vi "Run Caliper.vi"(6 "SelectionList":T3[](array[typedef]), 8 "error in (no error)":errorcluster, 9 "FilteredCaliperEntry":T6[](array[typedef]) {"CaliperType" items=["Distance", "Mid Point", "Perpendicular Projection", "Lines Intersection", "Angle from Horizontal", "Angle from Vertical", "Angle Defined by 3 Points", "Angle Defined by 4 Points", "Bissecting Line", "Mid Line", "Center of Mass", "Area", "Line Fit", "Circle Fit", "Ellipse Fit"]}, 10 "Analysis_Point_Result":T8[](array[typedef]), 11 "CaliperType":T2 items=["Distance", "Mid Point", "Perpendicular Projection", "Lines Intersection", "Angle from Horizontal", "Angle from Vertical", "Angle Defined by 3 Points", "Angle Defined by 4 Points", "Bissecting Line", "Mid Line", "Area", "Line Fit", "Circle Fit"]) -> (0 "error out":errorcluster, 2 "SelectionListOut":T3[](array[typedef]), 3 "Result":T5)   [LabVIEW 2019]
uses:
  Controls/CaliperType.ctl
  Controls/SelectionListEntry.ctl
  Controls/SelectionListEntryPointType.ctl
  Analysis/Controls/Analysis_Result_To_Caliper.ctl
  Controls/CaliperDataEntry_SinglePoint.ctl
  Controls/CaliperResult_SinglePoint.ctl
  Controls/CaliperResult.ctl
  Controls/CaliperDataEntry.ctl
  <vilib>/vision/NI_Vision_Development_Module.lvlib
panel:
  in  "CaliperEntry 2":T1 {"CaliperType" items=["Distance", "Mid Point", "Perpendicular Projection", "Lines Intersection", "Angle from Horizontal", "Angle from Vertical", "Angle Defined by 3 Points", "Angle Defined by 4 Points", "Bissecting Line", "Mid Line", "Center of Mass", "Area", "Line Fit", "Circle Fit", "Ellipse Fit"]}
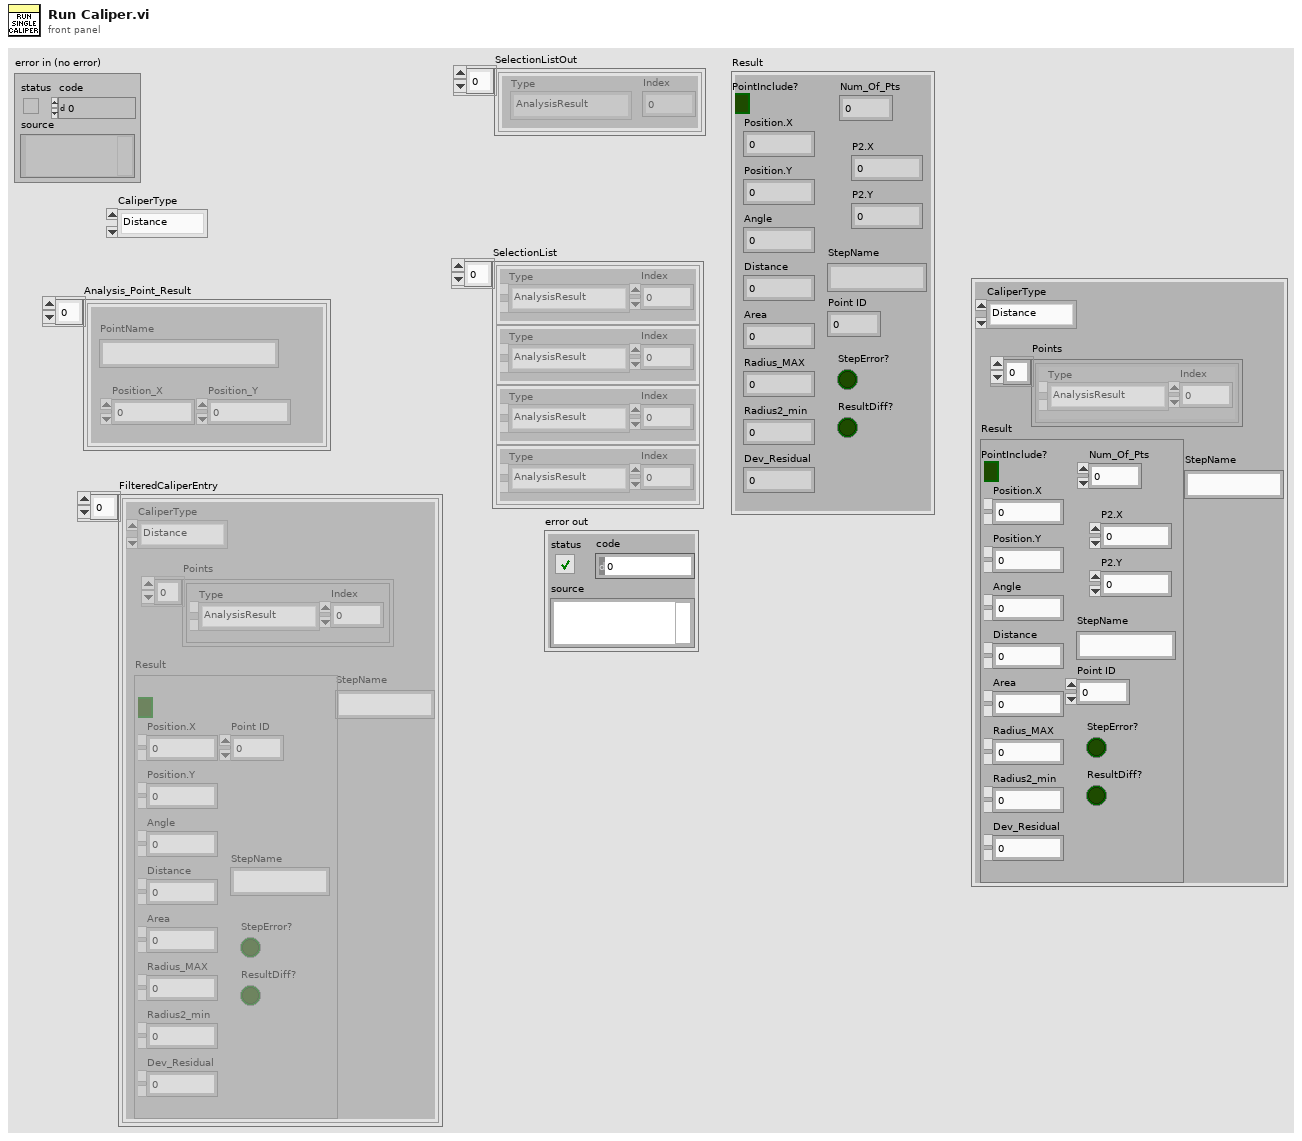
[diagram p1: front panel]
types:
  T1 = typedef "CaliperDataEntry.ctl" = cluster{"CaliperType":T2, "Points":T3[], "Result":T5, "StepName":string}
  T2 = typedef "CaliperType.ctl" = u32
  T3 = typedef "SelectionListEntry.ctl" = cluster{"Type":T4, "Index":i32}
  T4 = typedef "SelectionListEntryPointType.ctl" = enum16{"AnalysisResult", "CaliperResult"}
  T5 = typedef "CaliperResult.ctl" = cluster{"PointInclude?":bool, "Num_Of_Pts":u8, "Position.X":dbl, "Position.Y":dbl, "Angle":dbl, "Distance":dbl, "Area":dbl, "Radius_MAX":dbl, "Radius2_min":dbl, "Dev_Residual":dbl, "P2.X":dbl, "P2.Y":dbl, "StepName":string, "Point ID":u8, "StepError?":bool, "ResultDiff?":bool}
  T6 = typedef "CaliperDataEntry_SinglePoint.ctl" = cluster{"CaliperType":T2, "Points":T3[], "Result":T7, "StepName":string}
  T7 = typedef "CaliperResult_SinglePoint.ctl" = cluster{"PointInclude?":bool, "Position.X":dbl, "Position.Y":dbl, "Angle":dbl, "Distance":dbl, "Area":dbl, "Radius_MAX":dbl, "Radius2_min":dbl, "Dev_Residual":dbl, "StepName":string, "Point ID":u8, "StepError?":bool, "ResultDiff?":bool}
  T8 = typedef "Analysis_Result_To_Caliper.ctl" = cluster{"PointName":string, "Position_X":dbl, "Position_Y":dbl}
  T9 = cluster{cluster{"Position.X":dbl, "Position.Y":dbl}, cluster{"Position.X":dbl, "Position.Y":dbl}}
  T10 = cluster{"Point 1":cluster{"X":sgl, "Y":sgl}, "Point 2":cluster{"X":sgl, "Y":sgl}}
  T11 = cluster{"element":cluster{"Position_X":dbl, "Position_Y":dbl}, "element":cluster{"Position_X":dbl, "Position_Y":dbl}}
  T12 = cluster{"Center":cluster{"X":sgl, "Y":sgl}, "Radius":dbl}
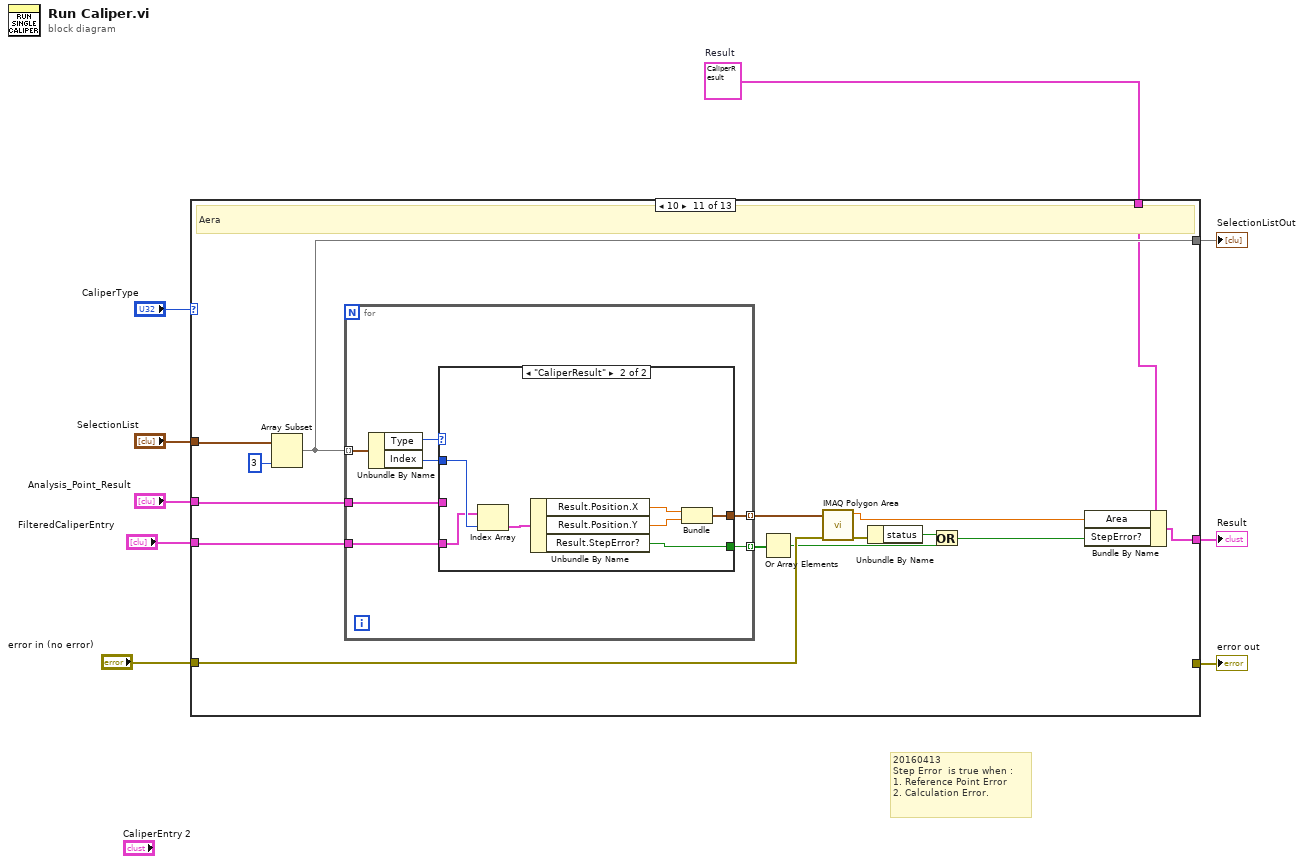
[diagram p0: block diagram]
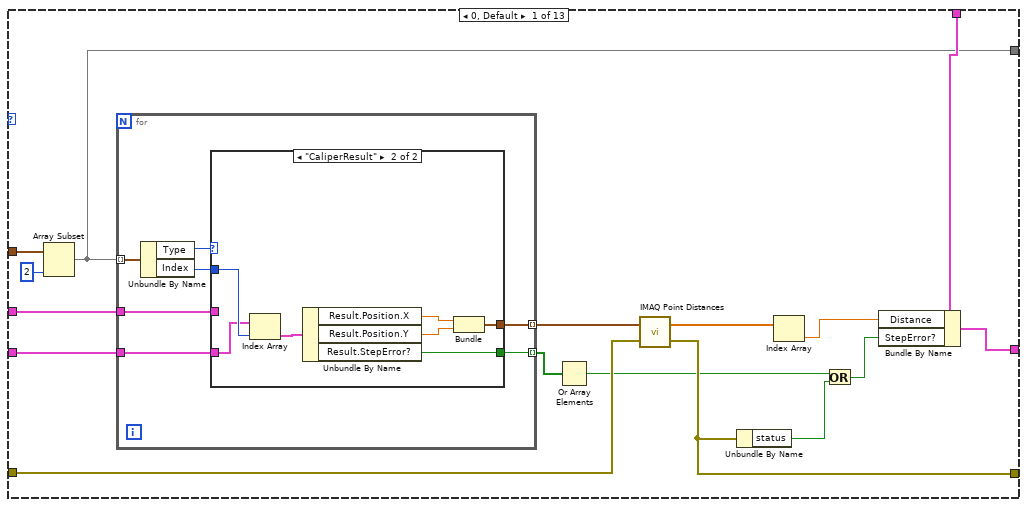
[diagram p2: hidden frame]
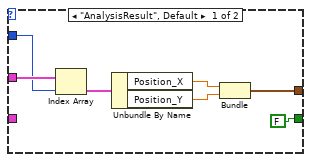
[diagram p3: hidden frame]
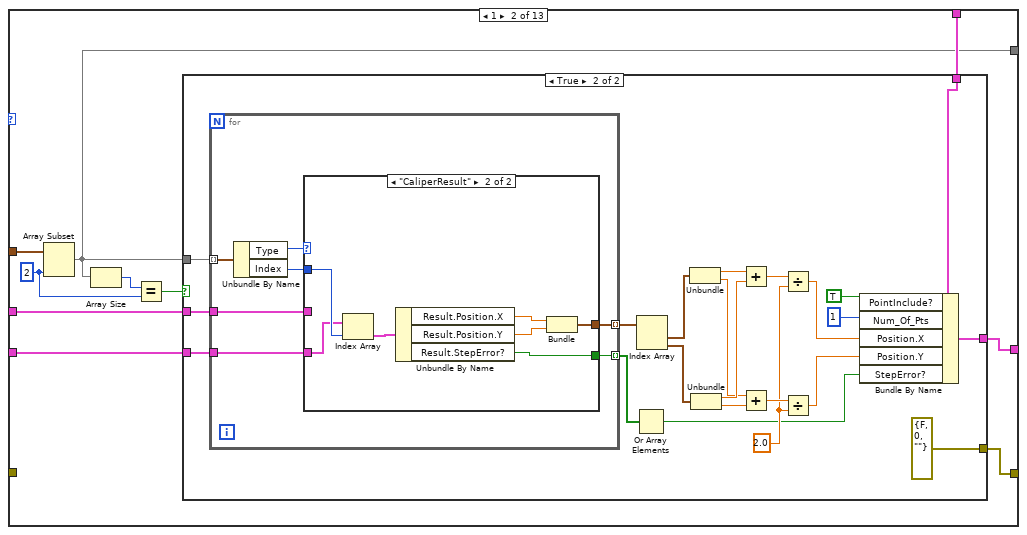
[diagram p4: hidden frame]
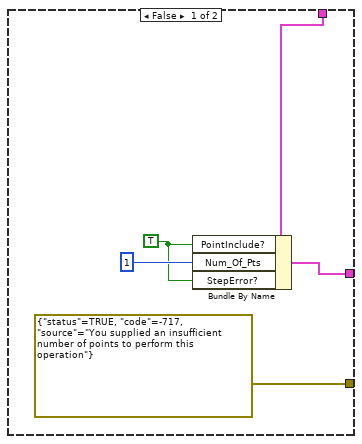
[diagram p5: hidden frame]
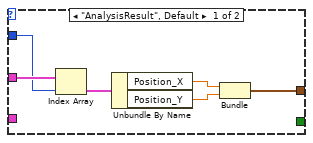
[diagram p6: hidden frame]
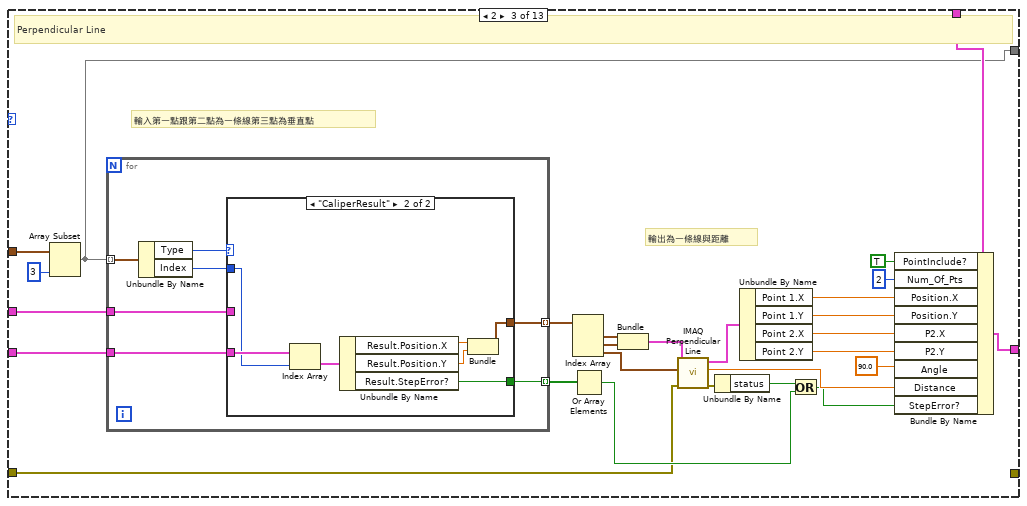
[diagram p7: hidden frame]
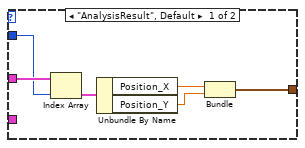
[diagram p8: hidden frame]
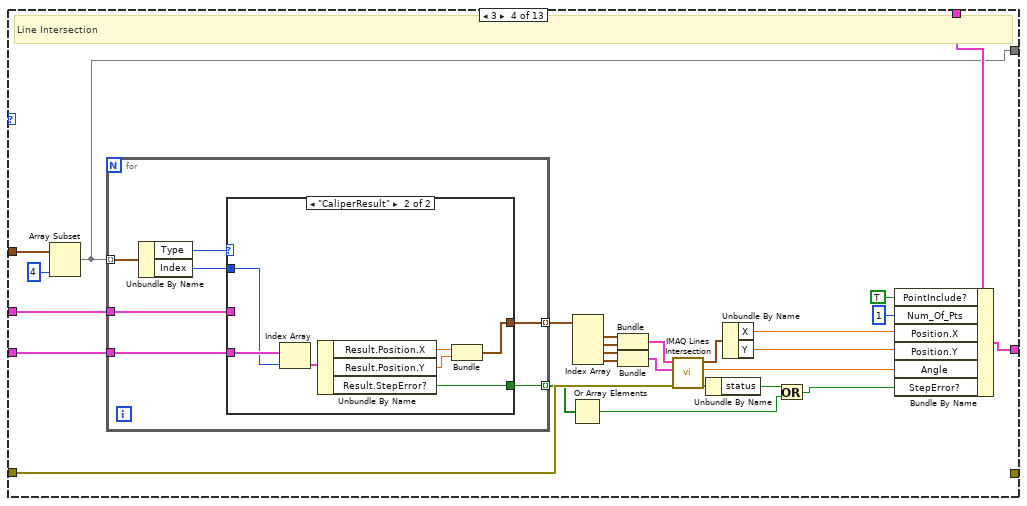
[diagram p9: hidden frame]
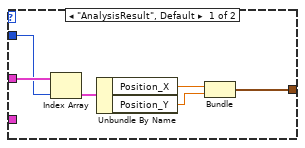
[diagram p10: hidden frame]
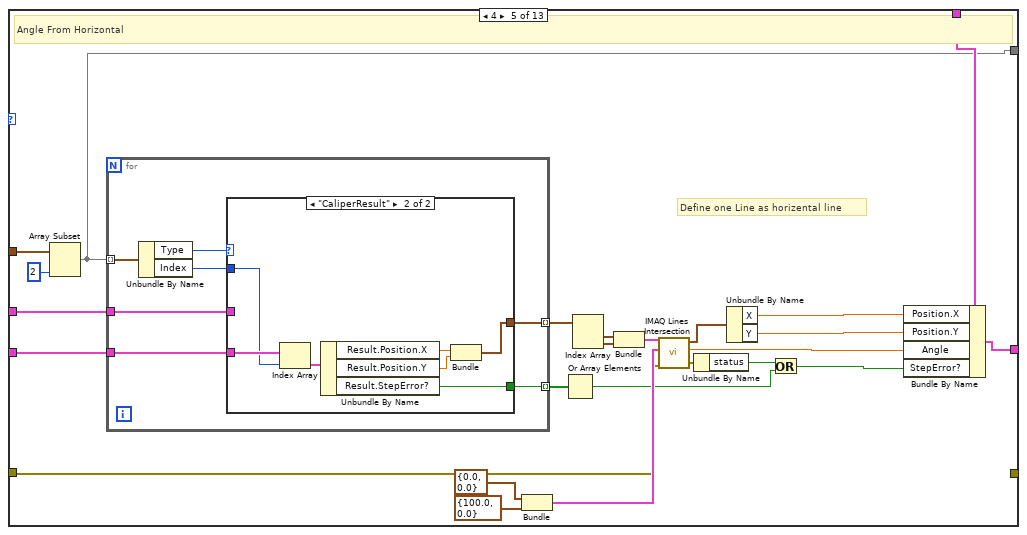
[diagram p11: hidden frame]
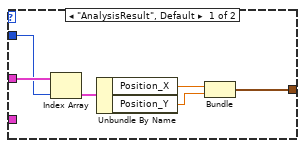
[diagram p12: hidden frame]
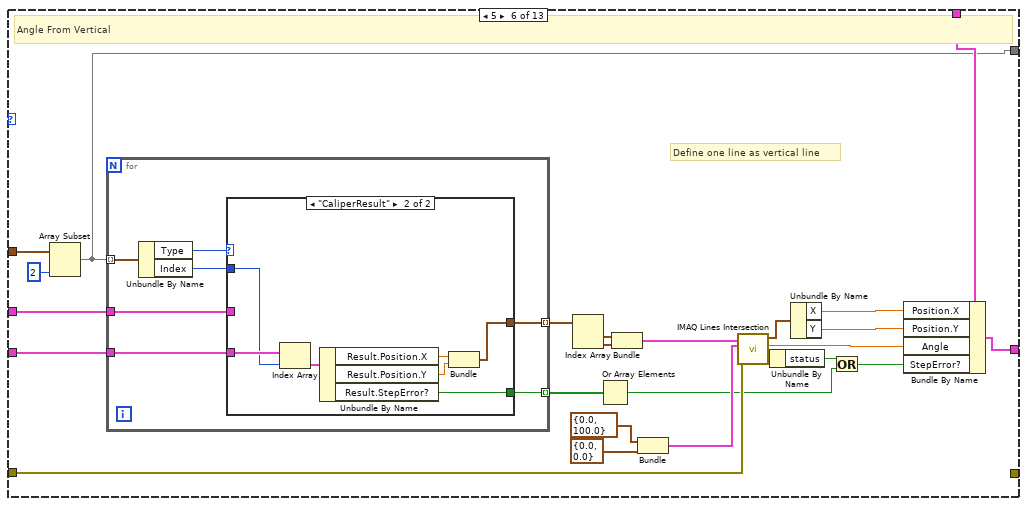
[diagram p13: hidden frame]
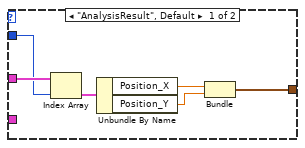
[diagram p14: hidden frame]
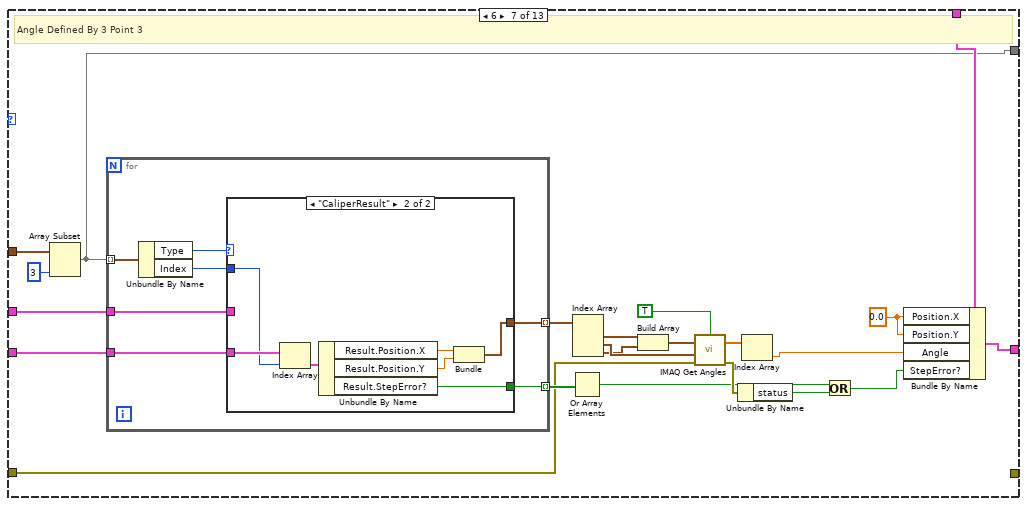
[diagram p15: hidden frame]
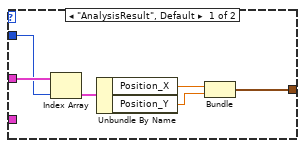
[diagram p16: hidden frame]
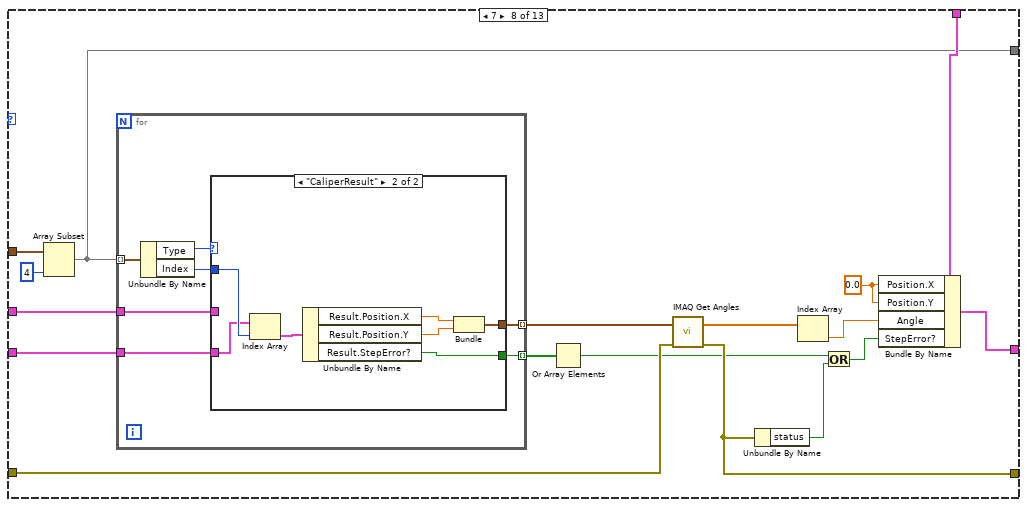
[diagram p17: hidden frame]
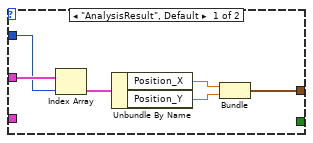
[diagram p18: hidden frame]
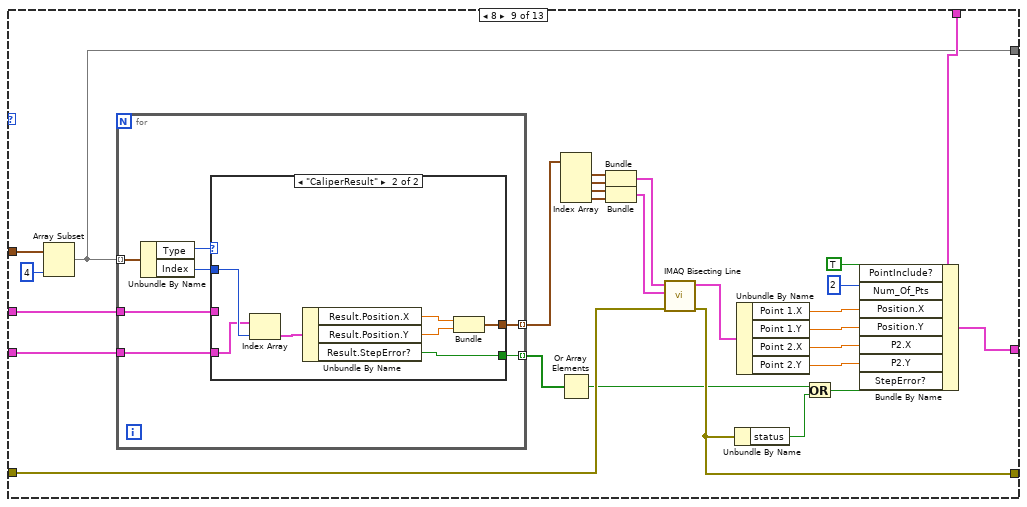
[diagram p19: hidden frame]
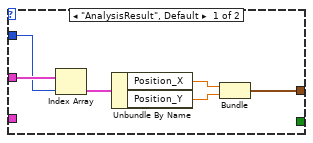
[diagram p20: hidden frame]
diagram:
  w6 = T5 {"PointInclude?"=FALSE, "Num_Of_Pts"=0, "Position.X"=0.0, "Position.Y"=0.0, "Angle"=0.0, "Distance"=0.0, "Area"=0.0, "Radius_MAX"=0.0, "Radius2_min"=0.0, "Dev_Residual"=0.0, "P2.X"=0.0, "P2.Y"=0.0, "StepName"="", "Point ID"=0, "StepError?"=FALSE, "ResultDiff?"=FALSE}  # Result
  # "20160413\nStep Error  is true when : \n1. Reference Point Error\n2. Calculation Error."
  n1 = case shown="10" "CaliperType" {
    tunnel: "SelectionList" -> [w25 w56 w130 w176 w220 w264 w306 w343 w390 w434 w469 w508 w547]
    tunnel: "Analysis_Point_Result" -> [w23 w53 w128 w174 w218 w262 w304 w341 w389 w433 w468 w507 w549]
    tunnel: w6 -> [w22 w54 w121 w169 w216 w259 w301 w340 w388 w424 w464 w501 w544]
    tunnel: [w19 w55 w120 w168 w215 w258 w300 w338 w387 w423 w462 w500 w543] -> w1
    tunnel: [w17 w51 w105 w151 w200 w244 w286 w337 w386 w431 w466 w505 w546] -> w5
    tunnel: [w14 w47 _ _ _ _ _ w332 w368 _ _ _ _] -> w3
    tunnel: "error in (no error)" -> [w16 _ w107 w157 w205 w249 w291 w334 w383 w415 w460 w493 w533]
    tunnel: "FilteredCaliperEntry" -> [w15 w52 w127 w173 w217 w261 w303 w336 w385 w432 w467 w506 w548]
    frame 0, Default {
      n2 = Array Subset(array=w25, length=2) -> (w17:T3[])  [unwired: 1 in]
      n3 = for {
        tunnel: w17 -> [w32] mode=indexing
        tunnel: w23 -> [w30]
        tunnel: [w28] -> w18 mode=indexing
        tunnel: w15 -> [w27]
        tunnel: [w26] -> w13 mode=indexing
        n4 = Unbundle By Name(w32) -> ("Type"=w31:T4, "Index"=w29:i32)
        n5 = case shown="\"CaliperResult\"" w31 {
          tunnel: w30 -> [w39 _]
          tunnel: w29 -> [w38 w46]
          tunnel: [w34 w42] -> w28
          tunnel: w27 -> [_ w41]
          tunnel: [FALSE ("StepError?") w40] -> w26
          frame "AnalysisResult", Default {
            n6 = Index Array(array=w39, index=w38) -> (element=w37:T8)
            n7 = Unbundle By Name(w37) -> ("Position_X"=w36:dbl, "Position_Y"=w35:dbl)
            n8 = Bundle("Position_X"=w36, "Position_Y"=w35) -> (w34:cluster{"Position_X":dbl, "Position_Y":dbl})  [unwired: 1 in]
          }
          frame "CaliperResult" {
            n9 = Index Array(array=w41, index=w46) -> (element=w45:T6)
            n10 = Unbundle By Name(w45) -> ("Result.Position.X"=w44:dbl, "Result.Position.Y"=w43:dbl, "Result.StepError?"=w40:bool)
            n11 = Bundle("Position.X"=w44, "Position.Y"=w43) -> (w42:cluster{"Position.X":dbl, "Position.Y":dbl})  [unwired: 1 in]
          }
        }
      }
      n12 = Or Array Elements(Boolean array=w13) -> (logical OR=w11:bool)
      n13 = call "IMAQ Point Distances"("Points"=w18, "error in (no error)"=w16) -> ("Distances"=w21:sgl[], "error out"=w14:errorcluster)  [unwired: 3 in]
      n14 = Unbundle By Name(w14) -> ("status"=w12:bool)
      n15 = Index Array(array=w21) -> (element=w20:sgl)  [unwired: 1 in]
      n16 = Or(x=w11, y=w12) -> (x .or. y?=w10:bool)
      n17 = Bundle By Name(cluster=w22, "Distance"=w20, "StepError?"=w10) -> (w19:T5)
    }
    frame 1 {
      w49 = 2 ("length")
      n18 = Array Subset(array=w56, length=w49) -> (w51:T3[])  [unwired: 1 in]
      n19 = Array Size(array=w51) -> (size(s)=w50:i32)
      n20 = Equal?(x=w50, y=w49) -> (x = y?=w48:bool)
      n21 = case shown="True" w48 {
        tunnel: [w58 w73] -> w55
        tunnel: w54 -> [w59 w72]
        tunnel: w53 -> [_ w69]
        tunnel: w51 -> [_ w67]
        tunnel: w52 -> [_ w66]
        tunnel: [errorcluster {"status"=TRUE, "code"=-717, "source"="You supplied an insufficient number of points to perform this operation"} ("error out") errorcluster {"status"=FALSE, "code"=0, "source"=""} ("error out")] -> w47
        frame False {
          w57 = TRUE ("PointInclude?")
          n22 = Bundle By Name(cluster=w59, "PointInclude?"=w57, "Num_Of_Pts"=u8 1, "StepError?"=w57) -> (w58:T5)
        }
        frame True {
          w76 = 2.0 ("y")
          n23 = for {
            tunnel: w67 -> [w90] mode=indexing
            tunnel: w69 -> [w88]
            tunnel: [w86] -> w68 mode=indexing
            tunnel: w66 -> [w85]
            tunnel: [w84] -> w63 mode=indexing
            n24 = Unbundle By Name(w90) -> ("Type"=w89:T4, "Index"=w87:i32)
            n25 = case shown="\"CaliperResult\"" w89 {
              tunnel: w88 -> [w96 _]
              tunnel: w87 -> [w95 w103]
              tunnel: [w91 w99] -> w86
              tunnel: w85 -> [_ w98]
              tunnel: [_ w97] -> w84
              frame "AnalysisResult", Default {
                n26 = Index Array(array=w96, index=w95) -> (element=w94:T8)
                n27 = Unbundle By Name(w94) -> ("Position_X"=w93:dbl, "Position_Y"=w92:dbl)
                n28 = Bundle("Position_X"=w93, "Position_Y"=w92) -> (w91:cluster{"Position_X":dbl, "Position_Y":dbl})  [unwired: 1 in]
              }
              frame "CaliperResult" {
                n29 = Index Array(array=w98, index=w103) -> (element=w102:T6)
                n30 = Unbundle By Name(w102) -> ("Result.Position.X"=w101:dbl, "Result.Position.Y"=w100:dbl, "Result.StepError?"=w97:bool)
                n31 = Bundle("Position.X"=w101, "Position.Y"=w100) -> (w99:cluster{"Position.X":dbl, "Position.Y":dbl})  [unwired: 1 in]
              }
            }
          }
          n32 = Or Array Elements(Boolean array=w63) -> (logical OR=w62:bool)
          n33 = Index Array(array=w68) -> (element #1=w83:cluster{"Position.X":dbl, "Position.Y":dbl}, element #2=w71:cluster{"Position.X":dbl, "Position.Y":dbl})  [unwired: 2 in]
          n34 = Unbundle(w83) -> ("Position.X"=w82:dbl, "Position.Y"=w79:dbl)
          n35 = Unbundle(w71) -> ("Position.X"=w80:dbl, "Position.Y"=w81:dbl)
          n36 = Add(x=w82, y=w80) -> (x+y=w78:dbl)
          n37 = Add(x=w79, y=w81) -> (x+y=w77:dbl)
          n38 = Divide(x=w78, y=w76) -> (x/y=w75:dbl)
          n39 = Divide(x=w77, y=w76) -> (x/y=w74:dbl)
          n40 = Bundle By Name(cluster=w72, "PointInclude?"=TRUE, "Num_Of_Pts"=u8 1, "Position.X"=w75, "Position.Y"=w74, "StepError?"=w62) -> (w73:T5)
        }
      }
    }
    frame 2 {
      # "輸出為一條線與距離"
      # "輸入第一點跟第二點為一條線第三點為垂直點"
      # "Perpendicular Line"
      n41 = Array Subset(array=w130, length=3) -> (w105:T3[])  [unwired: 1 in]
      n42 = for {
        tunnel: w105 -> [w137] mode=indexing
        tunnel: w128 -> [w135]
        tunnel: w127 -> [w132]
        tunnel: [w133] -> w126 mode=indexing
        tunnel: [w131] -> w111 mode=indexing
        n43 = Unbundle By Name(w137) -> ("Type"=w136:T4, "Index"=w134:i32)
        n44 = case shown="\"CaliperResult\"" w136 {
          tunnel: w135 -> [w143 _]
          tunnel: w134 -> [w142 w149]
          tunnel: [w138 w144] -> w133
          tunnel: w132 -> [_ w150]
          tunnel: [_ w147] -> w131
          frame "AnalysisResult", Default {
            n45 = Index Array(array=w143, index=w142) -> (element=w141:T8)
            n46 = Unbundle By Name(w141) -> ("Position_X"=w140:dbl, "Position_Y"=w139:dbl)
            n47 = Bundle("Position_X"=w140, "Position_Y"=w139) -> (w138:cluster{"Position_X":dbl, "Position_Y":dbl})  [unwired: 1 in]
          }
          frame "CaliperResult" {
            n48 = Index Array(array=w150, index=w149) -> (element=w148:T6)
            n49 = Unbundle By Name(w148) -> ("Result.Position.X"=w146:dbl, "Result.Position.Y"=w145:dbl, "Result.StepError?"=w147:bool)
            n50 = Bundle("Position.X"=w146, "Position.Y"=w145) -> (w144:cluster{"Position.X":dbl, "Position.Y":dbl})  [unwired: 1 in]
          }
        }
      }
      n51 = Index Array(array=w126) -> (element #1=w125:cluster{"Position.X":dbl, "Position.Y":dbl}, element #2=w124:cluster{"Position.X":dbl, "Position.Y":dbl}, element #3=w122:cluster{"Position.X":dbl, "Position.Y":dbl})  [unwired: 3 in]
      n52 = Or Array Elements(Boolean array=w111) -> (logical OR=w108:bool)
      n53 = Bundle(w125, w124) -> (w123:T9)  [unwired: 1 in]
      n54 = call "IMAQ Perpendicular Line"("error in (no error)"=w107, "Point"=w122, "Line"=w123) -> ("error out"=w110:errorcluster, "Distance"=w116:dbl, "Perpendicular Line"=w119:T10)  [unwired: 6 in]
      n55 = Unbundle By Name(w110) -> ("status"=w109:bool)
      n56 = Unbundle By Name(w119) -> ("Point 1.X"=w115:sgl, "Point 1.Y"=w114:sgl, "Point 2.X"=w118:sgl, "Point 2.Y"=w117:sgl)
      n57 = Or(x=w109, y=w108) -> (x .or. y?=w106:bool)
      n58 = Bundle By Name(cluster=w121, "PointInclude?"=TRUE, "Num_Of_Pts"=u8 2, "Position.X"=w115, "Position.Y"=w114, "P2.X"=w118, "P2.Y"=w117, "Angle"=90.0, "Distance"=w116, "StepError?"=w106) -> (w120:T5)
    }
    frame 3 {
      # "Line Intersection"
      n59 = Array Subset(array=w176, length=4) -> (w151:T3[])  [unwired: 1 in]
      n60 = for {
        tunnel: w151 -> [w183] mode=indexing
        tunnel: w174 -> [w181]
        tunnel: w173 -> [w178]
        tunnel: [w179] -> w172 mode=indexing
        tunnel: [w177] -> w156 mode=indexing
        n61 = Unbundle By Name(w183) -> ("Type"=w182:T4, "Index"=w180:i32)
        n62 = case shown="\"CaliperResult\"" w182 {
          tunnel: w181 -> [w189 _]
          tunnel: w180 -> [w188 w195]
          tunnel: [w184 w191] -> w179
          tunnel: w178 -> [_ w196]
          tunnel: [_ w190] -> w177
          frame "AnalysisResult", Default {
            n63 = Index Array(array=w189, index=w188) -> (element=w187:T8)
            n64 = Unbundle By Name(w187) -> ("Position_X"=w186:dbl, "Position_Y"=w185:dbl)
            n65 = Bundle("Position_X"=w186, "Position_Y"=w185) -> (w184:cluster{"Position_X":dbl, "Position_Y":dbl})  [unwired: 1 in]
          }
          frame "CaliperResult" {
            n66 = Index Array(array=w196, index=w195) -> (element=w194:T6)
            n67 = Unbundle By Name(w194) -> ("Result.Position.X"=w193:dbl, "Result.Position.Y"=w192:dbl, "Result.StepError?"=w190:bool)
            n68 = Bundle("Position.X"=w193, "Position.Y"=w192) -> (w191:cluster{"Position.X":dbl, "Position.Y":dbl})  [unwired: 1 in]
          }
        }
      }
      n69 = Or Array Elements(Boolean array=w156) -> (logical OR=w153:bool)
      n70 = Index Array(array=w172) -> (element #1=w171:cluster{"Position.X":dbl, "Position.Y":dbl}, element #2=w170:cluster{"Position.X":dbl, "Position.Y":dbl}, element #3=w167:cluster{"Position.X":dbl, "Position.Y":dbl}, element #4=w166:cluster{"Position.X":dbl, "Position.Y":dbl})  [unwired: 4 in]
      n71 = Bundle(w171, w170) -> (w165:T9)  [unwired: 1 in]
      n72 = Bundle(w167, w166) -> (w164:T9)  [unwired: 1 in]
      n73 = call "IMAQ Lines Intersection"("error in (no error)"=w157, "Line 2"=w164, "Line 1"=w165) -> ("error out"=w155:errorcluster, "Angle"=w160:dbl, "Intersection Point"=w163:cluster{"X":sgl, "Y":sgl})  [unwired: 6 in]
      n74 = Unbundle By Name(w155) -> ("status"=w154:bool)
      n75 = Unbundle By Name(w163) -> ("X"=w162:sgl, "Y"=w161:sgl)
      n76 = Or(x=w154, y=w153) -> (x .or. y?=w152:bool)
      n77 = Bundle By Name(cluster=w169, "PointInclude?"=TRUE, "Num_Of_Pts"=u8 1, "Position.X"=w162, "Position.Y"=w161, "Angle"=w160, "StepError?"=w152) -> (w168:T5)
    }
    frame 4 {
      # "Define one Line as horizental line"
      # "Angle From Horizontal"
      n78 = Array Subset(array=w220, length=2) -> (w200:T3[])  [unwired: 1 in]
      n79 = for {
        tunnel: w200 -> [w227] mode=indexing
        tunnel: w218 -> [w225]
        tunnel: w217 -> [w222]
        tunnel: [w223] -> w209 mode=indexing
        tunnel: [w221] -> w206 mode=indexing
        n80 = Unbundle By Name(w227) -> ("Type"=w226:T4, "Index"=w224:i32)
        n81 = case shown="\"CaliperResult\"" w226 {
          tunnel: w225 -> [w233 _]
          tunnel: w224 -> [w232 w239]
          tunnel: [w228 w235] -> w223
          tunnel: w222 -> [_ w240]
          tunnel: [_ w234] -> w221
          frame "AnalysisResult", Default {
            n82 = Index Array(array=w233, index=w232) -> (element=w231:T8)
            n83 = Unbundle By Name(w231) -> ("Position_X"=w230:dbl, "Position_Y"=w229:dbl)
            n84 = Bundle("Position_X"=w230, "Position_Y"=w229) -> (w228:cluster{"Position_X":dbl, "Position_Y":dbl})  [unwired: 1 in]
          }
          frame "CaliperResult" {
            n85 = Index Array(array=w240, index=w239) -> (element=w238:T6)
            n86 = Unbundle By Name(w238) -> ("Result.Position.X"=w237:dbl, "Result.Position.Y"=w236:dbl, "Result.StepError?"=w234:bool)
            n87 = Bundle("Position.X"=w237, "Position.Y"=w236) -> (w235:cluster{"Position.X":dbl, "Position.Y":dbl})  [unwired: 1 in]
          }
        }
      }
      n88 = Bundle("element"=cluster{"Position_X":dbl, "Position_Y":dbl} {"Position_X"=0.0, "Position_Y"=0.0}, "element"=cluster{"Position_X":dbl, "Position_Y":dbl} {"Position_X"=100.0, "Position_Y"=0.0}) -> (w210:T11)  [unwired: 1 in]
      n89 = Or Array Elements(Boolean array=w206) -> (logical OR=w202:bool)
      n90 = Index Array(array=w209) -> (element #1=w214:cluster{"Position.X":dbl, "Position.Y":dbl}, element #2=w213:cluster{"Position.X":dbl, "Position.Y":dbl})  [unwired: 2 in]
      n91 = Bundle(w214, w213) -> (w212:T9)  [unwired: 1 in]
      n92 = call "IMAQ Lines Intersection"("error in (no error)"=w205, "Line 2"=w210, "Line 1"=w212) -> ("error out"=w204:errorcluster, "Angle"=w208:dbl, "Intersection Point"=w199:cluster{"X":sgl, "Y":sgl})  [unwired: 6 in]
      n93 = Unbundle By Name(w204) -> ("status"=w203:bool)
      n94 = Unbundle By Name(w199) -> ("X"=w198:sgl, "Y"=w197:sgl)
      n95 = Or(x=w203, y=w202) -> (x .or. y?=w201:bool)
      n96 = Bundle By Name(cluster=w216, "Position.X"=w198, "Position.Y"=w197, "Angle"=w208, "StepError?"=w201) -> (w215:T5)
    }
    frame 5 {
      # "Define one line as vertical line"
      # "Angle From Vertical"
      n97 = Array Subset(array=w264, length=2) -> (w244:T3[])  [unwired: 1 in]
      n98 = for {
        tunnel: w244 -> [w271] mode=indexing
        tunnel: w262 -> [w269]
        tunnel: w261 -> [w266]
        tunnel: [w267] -> w260 mode=indexing
        tunnel: [w265] -> w250 mode=indexing
        n99 = Unbundle By Name(w271) -> ("Type"=w270:T4, "Index"=w268:i32)
        n100 = case shown="\"CaliperResult\"" w270 {
          tunnel: w269 -> [w277 _]
          tunnel: w268 -> [w276 w283]
          tunnel: [w272 w279] -> w267
          tunnel: w266 -> [_ w284]
          tunnel: [_ w278] -> w265
          frame "AnalysisResult", Default {
            n101 = Index Array(array=w277, index=w276) -> (element=w275:T8)
            n102 = Unbundle By Name(w275) -> ("Position_X"=w274:dbl, "Position_Y"=w273:dbl)
            n103 = Bundle("Position_X"=w274, "Position_Y"=w273) -> (w272:cluster{"Position_X":dbl, "Position_Y":dbl})  [unwired: 1 in]
          }
          frame "CaliperResult" {
            n104 = Index Array(array=w284, index=w283) -> (element=w282:T6)
            n105 = Unbundle By Name(w282) -> ("Result.Position.X"=w281:dbl, "Result.Position.Y"=w280:dbl, "Result.StepError?"=w278:bool)
            n106 = Bundle("Position.X"=w281, "Position.Y"=w280) -> (w279:cluster{"Position.X":dbl, "Position.Y":dbl})  [unwired: 1 in]
          }
        }
      }
      n107 = Index Array(array=w260) -> (element #1=w257:cluster{"Position.X":dbl, "Position.Y":dbl}, element #2=w256:cluster{"Position.X":dbl, "Position.Y":dbl})  [unwired: 2 in]
      n108 = Or Array Elements(Boolean array=w250) -> (logical OR=w246:bool)
      n109 = Bundle(w257, w256) -> (w255:T9)  [unwired: 1 in]
      n110 = Bundle("element"=cluster{"Position_X":dbl, "Position_Y":dbl} {"Position_X"=0.0, "Position_Y"=100.0}, "element"=cluster{"Position_X":dbl, "Position_Y":dbl} {"Position_X"=0.0, "Position_Y"=0.0}) -> (w251:T11)  [unwired: 1 in]
      n111 = call "IMAQ Lines Intersection"("error in (no error)"=w249, "Line 2"=w251, "Line 1"=w255) -> ("error out"=w248:errorcluster, "Angle"=w254:dbl, "Intersection Point"=w243:cluster{"X":sgl, "Y":sgl})  [unwired: 6 in]
      n112 = Unbundle By Name(w248) -> ("status"=w247:bool)
      n113 = Unbundle By Name(w243) -> ("X"=w242:sgl, "Y"=w241:sgl)
      n114 = Or(x=w247, y=w246) -> (x .or. y?=w245:bool)
      n115 = Bundle By Name(cluster=w259, "Position.X"=w242, "Position.Y"=w241, "Angle"=w254, "StepError?"=w245) -> (w258:T5)
    }
    frame 6 {
      w285 = 0.0 ("Position.X")
      # "Angle Defined By 3 Point 3"
      n116 = Array Subset(array=w306, length=3) -> (w286:T3[])  [unwired: 1 in]
      n117 = for {
        tunnel: w286 -> [w313] mode=indexing
        tunnel: w304 -> [w311]
        tunnel: w303 -> [w308]
        tunnel: [w309] -> w302 mode=indexing
        tunnel: [w307] -> w292 mode=indexing
        n118 = Unbundle By Name(w313) -> ("Type"=w312:T4, "Index"=w310:i32)
        n119 = case shown="\"CaliperResult\"" w312 {
          tunnel: w311 -> [w319 _]
          tunnel: w310 -> [w318 w325]
          tunnel: [w314 w321] -> w309
          tunnel: w308 -> [_ w326]
          tunnel: [_ w320] -> w307
          frame "AnalysisResult", Default {
            n120 = Index Array(array=w319, index=w318) -> (element=w317:T8)
            n121 = Unbundle By Name(w317) -> ("Position_X"=w316:dbl, "Position_Y"=w315:dbl)
            n122 = Bundle("Position_X"=w316, "Position_Y"=w315) -> (w314:cluster{"Position_X":dbl, "Position_Y":dbl})  [unwired: 1 in]
          }
          frame "CaliperResult" {
            n123 = Index Array(array=w326, index=w325) -> (element=w324:T6)
            n124 = Unbundle By Name(w324) -> ("Result.Position.X"=w323:dbl, "Result.Position.Y"=w322:dbl, "Result.StepError?"=w320:bool)
            n125 = Bundle("Position.X"=w323, "Position.Y"=w322) -> (w321:cluster{"Position.X":dbl, "Position.Y":dbl})  [unwired: 1 in]
          }
        }
      }
      n126 = Or Array Elements(Boolean array=w292) -> (logical OR=w289:bool)
      n127 = Index Array(array=w302) -> (element #1=w298:cluster{"Position.X":dbl, "Position.Y":dbl}, element #2=w299:cluster{"Position.X":dbl, "Position.Y":dbl}, element #3=w297:cluster{"Position.X":dbl, "Position.Y":dbl})  [unwired: 3 in]
      n128 = Build Array(w298, w297) -> (w296:cluster{"Position.X":dbl, "Position.Y":dbl}[])
      n129 = call "IMAQ Get Angles"("error in (no error)"=w291, "Vertex"=w299, "Points"=w296, "Use Vertex (No)"=TRUE) -> ("error out"=w290:errorcluster, "Angles (deg)"=w295:sgl[])  [unwired: 1 in, 1 out]
      n130 = Unbundle By Name(w290) -> ("status"=w288:bool)
      n131 = Index Array(array=w295) -> (element=w294:sgl)  [unwired: 1 in]
      n132 = Or(x=w289, y=w288) -> (x .or. y?=w287:bool)
      n133 = Bundle By Name(cluster=w301, "Position.X"=w285, "Position.Y"=w285, "Angle"=w294, "StepError?"=w287) -> (w300:T5)
    }
    frame 7 {
      w327 = 0.0 ("Position.X")
      n134 = Array Subset(array=w343, length=4) -> (w337:T3[])  [unwired: 1 in]
      n135 = for {
        tunnel: w337 -> [w350] mode=indexing
        tunnel: w341 -> [w348]
        tunnel: [w346] -> w335 mode=indexing
        tunnel: w336 -> [w345]
        tunnel: [w344] -> w331 mode=indexing
        n136 = Unbundle By Name(w350) -> ("Type"=w349:T4, "Index"=w347:i32)
        n137 = case shown="\"CaliperResult\"" w349 {
          tunnel: w348 -> [w356 _]
          tunnel: w347 -> [w355 w363]
          tunnel: [w351 w359] -> w346
          tunnel: w345 -> [_ w358]
          tunnel: [_ w357] -> w344
          frame "AnalysisResult", Default {
            n138 = Index Array(array=w356, index=w355) -> (element=w354:T8)
            n139 = Unbundle By Name(w354) -> ("Position_X"=w353:dbl, "Position_Y"=w352:dbl)
            n140 = Bundle("Position_X"=w353, "Position_Y"=w352) -> (w351:cluster{"Position_X":dbl, "Position_Y":dbl})  [unwired: 1 in]
          }
          frame "CaliperResult" {
            n141 = Index Array(array=w358, index=w363) -> (element=w362:T6)
            n142 = Unbundle By Name(w362) -> ("Result.Position.X"=w361:dbl, "Result.Position.Y"=w360:dbl, "Result.StepError?"=w357:bool)
            n143 = Bundle("Position.X"=w361, "Position.Y"=w360) -> (w359:cluster{"Position.X":dbl, "Position.Y":dbl})  [unwired: 1 in]
          }
        }
      }
      n144 = Or Array Elements(Boolean array=w331) -> (logical OR=w330:bool)
      n145 = call "IMAQ Get Angles"("error in (no error)"=w334, "Points"=w335) -> ("error out"=w332:errorcluster, "Angles (deg)"=w333:sgl[])  [unwired: 3 in, 1 out]
      n146 = Unbundle By Name(w332) -> ("status"=w329:bool)
      n147 = Index Array(array=w333) -> (element=w339:sgl)  [unwired: 1 in]
      n148 = Or(x=w330, y=w329) -> (x .or. y?=w328:bool)
      n149 = Bundle By Name(cluster=w340, "Position.X"=w327, "Position.Y"=w327, "Angle"=w339, "StepError?"=w328) -> (w338:T5)
    }
    frame 8 {
      n150 = Array Subset(array=w390, length=4) -> (w386:T3[])  [unwired: 1 in]
      n151 = for {
        tunnel: w386 -> [w397] mode=indexing
        tunnel: w389 -> [w395]
        tunnel: [w393] -> w382 mode=indexing
        tunnel: w385 -> [w392]
        tunnel: [w391] -> w366 mode=indexing
        n152 = Unbundle By Name(w397) -> ("Type"=w396:T4, "Index"=w394:i32)
        n153 = case shown="\"CaliperResult\"" w396 {
          tunnel: w395 -> [w403 _]
          tunnel: w394 -> [w402 w410]
          tunnel: [w398 w406] -> w393
          tunnel: w392 -> [_ w405]
          tunnel: [_ w404] -> w391
          frame "AnalysisResult", Default {
            n154 = Index Array(array=w403, index=w402) -> (element=w401:T8)
            n155 = Unbundle By Name(w401) -> ("Position_X"=w400:dbl, "Position_Y"=w399:dbl)
            n156 = Bundle("Position_X"=w400, "Position_Y"=w399) -> (w398:cluster{"Position_X":dbl, "Position_Y":dbl})  [unwired: 1 in]
          }
          frame "CaliperResult" {
            n157 = Index Array(array=w405, index=w410) -> (element=w409:T6)
            n158 = Unbundle By Name(w409) -> ("Result.Position.X"=w408:dbl, "Result.Position.Y"=w407:dbl, "Result.StepError?"=w404:bool)
            n159 = Bundle("Position.X"=w408, "Position.Y"=w407) -> (w406:cluster{"Position.X":dbl, "Position.Y":dbl})  [unwired: 1 in]
          }
        }
      }
      n160 = Index Array(array=w382) -> (element #1=w381:cluster{"Position.X":dbl, "Position.Y":dbl}, element #2=w380:cluster{"Position.X":dbl, "Position.Y":dbl}, element #3=w379:cluster{"Position.X":dbl, "Position.Y":dbl}, element #4=w378:cluster{"Position.X":dbl, "Position.Y":dbl})  [unwired: 4 in]
      n161 = Or Array Elements(Boolean array=w366) -> (logical OR=w365:bool)
      n162 = Bundle(w381, w380) -> (w377:T9)  [unwired: 1 in]
      n163 = Bundle(w379, w378) -> (w376:T9)  [unwired: 1 in]
      n164 = call "IMAQ Bisecting Line"("error in (no error)"=w383, "Line 2"=w376, "Line 1"=w377) -> ("error out"=w368:errorcluster, "Bisecting Line"=w374:T10)  [unwired: 7 in]
      n165 = Unbundle By Name(w368) -> ("status"=w367:bool)
      n166 = Unbundle By Name(w374) -> ("Point 1.X"=w373:sgl, "Point 1.Y"=w372:sgl, "Point 2.X"=w371:sgl, "Point 2.Y"=w370:sgl)
      n167 = Or(x=w365, y=w367) -> (x .or. y?=w364:bool)
      n168 = Bundle By Name(cluster=w388, "PointInclude?"=TRUE, "Num_Of_Pts"=u8 2, "Position.X"=w373, "Position.Y"=w372, "P2.X"=w371, "P2.Y"=w370, "StepError?"=w364) -> (w387:T5)
    }
    frame 9 {
      # "輸出中線"
      # "輸入第一點與第二點為直線第三點為中點"
      # "Mid Line尋找點與線中間的中線"
      n169 = Array Subset(array=w434, length=3) -> (w431:T3[])  [unwired: 1 in]
      n170 = for {
        tunnel: w431 -> [w442] mode=indexing
        tunnel: w433 -> [w440]
        tunnel: [w438] -> w430 mode=indexing
        tunnel: w432 -> [w437]
        tunnel: [w436] -> w416 mode=indexing
        n171 = Unbundle By Name(w442) -> ("Type"=w441:T4, "Index"=w439:i32)
        n172 = case shown="\"AnalysisResult\", Default" w441 {
          tunnel: w440 -> [w448 _]
          tunnel: w439 -> [w447 w455]
          tunnel: [w443 w451] -> w438
          tunnel: w437 -> [_ w450]
          tunnel: [_ w449] -> w436
          frame "AnalysisResult", Default {
            n173 = Index Array(array=w448, index=w447) -> (element=w446:T8)
            n174 = Unbundle By Name(w446) -> ("Position_X"=w445:dbl, "Position_Y"=w444:dbl)
            n175 = Bundle("Position_X"=w445, "Position_Y"=w444) -> (w443:cluster{"Position_X":dbl, "Position_Y":dbl})  [unwired: 1 in]
          }
          frame "CaliperResult" {
            n176 = Index Array(array=w450, index=w455) -> (element=w454:T6)
            n177 = Unbundle By Name(w454) -> ("Result.Position.X"=w453:dbl, "Result.Position.Y"=w452:dbl, "Result.StepError?"=w449:bool)
            n178 = Bundle("Position.X"=w453, "Position.Y"=w452) -> (w451:cluster{"Position.X":dbl, "Position.Y":dbl})  [unwired: 1 in]
          }
        }
      }
      n179 = Or Array Elements(Boolean array=w416) -> (logical OR=w412:bool)
      n180 = Index Array(array=w430) -> (element #1=w429:cluster{"Position.X":dbl, "Position.Y":dbl}, element #2=w428:cluster{"Position.X":dbl, "Position.Y":dbl}, element #3=w426:cluster{"Position.X":dbl, "Position.Y":dbl})  [unwired: 3 in]
      n181 = Bundle(w429, w428) -> (w427:T9)  [unwired: 1 in]
      n182 = call "IMAQ Mid Line"("error in (no error)"=w415, "Point"=w426, "Line"=w427) -> ("error out"=w414:errorcluster, "Bisecting Line"=w425:T10)  [unwired: 7 in]
      n183 = Unbundle By Name(w414) -> ("status"=w413:bool)
      n184 = Unbundle By Name(w425) -> ("Point 1.X"=w422:sgl, "Point 1.Y"=w421:sgl, "Point 2.X"=w420:sgl, "Point 2.Y"=w419:sgl)
      n185 = Or(x=w413, y=w412) -> (x .or. y?=w411:bool)
      n186 = Bundle By Name(cluster=w424, "PointInclude?"=TRUE, "Num_Of_Pts"=u8 2, "Position.X"=w422, "Position.Y"=w421, "P2.X"=w420, "P2.Y"=w419, "StepError?"=w411) -> (w423:T5)
    }
    frame 10 {
      # "Aera"
      n187 = Array Subset(array=w469, length=3) -> (w466:T3[])  [unwired: 1 in]
      n188 = for {
        tunnel: w466 -> [w477] mode=indexing
        tunnel: w468 -> [w475]
        tunnel: [w473] -> w465 mode=indexing
        tunnel: w467 -> [w472]
        tunnel: [w471] -> w461 mode=indexing
        n189 = Unbundle By Name(w477) -> ("Type"=w476:T4, "Index"=w474:i32)
        n190 = case shown="\"CaliperResult\"" w476 {
          tunnel: w475 -> [w483 _]
          tunnel: w474 -> [w482 w490]
          tunnel: [w478 w486] -> w473
          tunnel: w472 -> [_ w485]
          tunnel: [_ w484] -> w471
          frame "AnalysisResult", Default {
            n191 = Index Array(array=w483, index=w482) -> (element=w481:T8)
            n192 = Unbundle By Name(w481) -> ("Position_X"=w480:dbl, "Position_Y"=w479:dbl)
            n193 = Bundle("Position_X"=w480, "Position_Y"=w479) -> (w478:cluster{"Position_X":dbl, "Position_Y":dbl})  [unwired: 1 in]
          }
          frame "CaliperResult" {
            n194 = Index Array(array=w485, index=w490) -> (element=w489:T6)
            n195 = Unbundle By Name(w489) -> ("Result.Position.X"=w488:dbl, "Result.Position.Y"=w487:dbl, "Result.StepError?"=w484:bool)
            n196 = Bundle("Position.X"=w488, "Position.Y"=w487) -> (w486:cluster{"Position.X":dbl, "Position.Y":dbl})  [unwired: 1 in]
          }
        }
      }
      n197 = Or Array Elements(Boolean array=w461) -> (logical OR=w457:bool)
      n198 = call "IMAQ Polygon Area"("error in (no error)"=w460, "Vertex Points"=w465) -> ("error out"=w459:errorcluster, "Area"=w463:sgl)  [unwired: 8 in]
      n199 = Unbundle By Name(w459) -> ("status"=w458:bool)
      n200 = Or(x=w458, y=w457) -> (x .or. y?=w456:bool)
      n201 = Bundle By Name(cluster=w464, "Area"=w463, "StepError?"=w456) -> (w462:T5)
    }
    frame 11 {
      # "Line Fit"
      n202 = Array Subset(array=w508, length=2) -> (w505:T3[])  [unwired: 1 in]
      n203 = for {
        tunnel: w505 -> [w516] mode=indexing
        tunnel: w507 -> [w514]
        tunnel: [w512] -> w504 mode=indexing
        tunnel: w506 -> [w511]
        tunnel: [w510] -> _ mode=indexing
        n204 = Unbundle By Name(w516) -> ("Type"=w515:T4, "Index"=w513:i32)
        n205 = case shown="\"AnalysisResult\", Default" w515 {
          tunnel: w514 -> [w522 _]
          tunnel: w513 -> [w521 w529]
          tunnel: [w517 w525] -> w512
          tunnel: w511 -> [_ w524]
          tunnel: [_ w523] -> w510
          frame "AnalysisResult", Default {
            n206 = Index Array(array=w522, index=w521) -> (element=w520:T8)
            n207 = Unbundle By Name(w520) -> ("Position_X"=w519:dbl, "Position_Y"=w518:dbl)
            n208 = Bundle("Position_X"=w519, "Position_Y"=w518) -> (w517:cluster{"Position_X":dbl, "Position_Y":dbl})  [unwired: 1 in]
          }
          frame "CaliperResult" {
            n209 = Index Array(array=w524, index=w529) -> (element=w528:T6)
            n210 = Unbundle By Name(w528) -> ("Result.Position.X"=w527:dbl, "Result.Position.Y"=w526:dbl, "Result.StepError?"=w523:bool)
            n211 = Bundle("Position.X"=w527, "Position.Y"=w526) -> (w525:cluster{"Position.X":dbl, "Position.Y":dbl})  [unwired: 1 in]
          }
        }
      }
      n212 = call "IMAQ Fit Line"("Points"=w504) -> ("error out"=w494:errorcluster, "Valid Fit?"=w492:bool, "Residual"=w495:dbl, "Line Segment"=w503:T10)  [unwired: 5 in, 2 out]
      n213 = Unbundle By Name(w503) -> ("Point 1.X"=w499:sgl, "Point 1.Y"=w498:sgl, "Point 2.X"=w497:sgl, "Point 2.Y"=w496:sgl)
      n214 = Compound Arithmetic op=OR(w494, w493, w492) -> (w491:bool)
      n215 = Bundle By Name(cluster=w501, "PointInclude?"=TRUE, "Position.X"=w499, "Position.Y"=w498, "P2.X"=w497, "P2.Y"=w496, "Radius_MAX"=w495, "StepError?"=w491) -> (w500:T5)
    }
    frame 12 {
      # "Circle Fit"
      n216 = Array Subset(array=w547, length=3) -> (w546:T3[])  [unwired: 1 in]
      n217 = for {
        tunnel: w546 -> [w557] mode=indexing
        tunnel: w549 -> [w555]
        tunnel: [w553] -> w545 mode=indexing
        tunnel: w548 -> [w552]
        tunnel: [w551] -> _ mode=indexing
        n218 = Unbundle By Name(w557) -> ("Type"=w556:T4, "Index"=w554:i32)
        n219 = case shown="\"AnalysisResult\", Default" w556 {
          tunnel: w555 -> [w563 _]
          tunnel: w554 -> [w562 w570]
          tunnel: [w558 w566] -> w553
          tunnel: w552 -> [_ w565]
          tunnel: [_ w564] -> w551
          frame "AnalysisResult", Default {
            n220 = Index Array(array=w563, index=w562) -> (element=w561:T8)
            n221 = Unbundle By Name(w561) -> ("Position_X"=w560:dbl, "Position_Y"=w559:dbl)
            n222 = Bundle("Position_X"=w560, "Position_Y"=w559) -> (w558:cluster{"Position_X":dbl, "Position_Y":dbl})  [unwired: 1 in]
          }
          frame "CaliperResult" {
            n223 = Index Array(array=w565, index=w570) -> (element=w569:T6)
            n224 = Unbundle By Name(w569) -> ("Result.Position.X"=w568:dbl, "Result.Position.Y"=w567:dbl, "Result.StepError?"=w564:bool)
            n225 = Bundle("Position.X"=w568, "Position.Y"=w567) -> (w566:cluster{"Position.X":dbl, "Position.Y":dbl})  [unwired: 1 in]
          }
        }
      }
      n226 = call "IMAQ Fit Circle 2"("Radial Points"=w545) -> ("error out"=w534:errorcluster, "Measurements"=w538:cluster{"Area":dbl, "Perimeter":dbl}, "Circle"=w542:T12)  [unwired: 5 in, 3 out]
      n227 = Unbundle By Name(w542) -> ("Center.X"=w541:sgl, "Center.Y"=w540:sgl, "Radius"=w536:dbl)
      n228 = Unbundle By Name(w538) -> ("Area"=w537:dbl, "Perimeter"=w535:dbl)
      n229 = Merge Errors(w534, w533) -> (w532:errorcluster)
      n230 = Unbundle By Name(w532) -> ("status"=w531:bool)
      n231 = Bundle By Name(cluster=w544, "PointInclude?"=TRUE, "Position.X"=w541, "Position.Y"=w540, "Distance"=w535, "Area"=w537, "Radius_MAX"=w536, "StepError?"=w531, "Num_Of_Pts"=u8 1) -> (w543:T5)
    }
  }
  "SelectionListOut" <- w5
  "error out" <- w3
  "Result" <- w1
